vi "ap2 (hw4).vi"() -> ()   [LabVIEW 2017]
panel:
  in  "Stop":bool
  out "Equation used":string
  out "Result":dbl
  in  "Operation":T1(ring)
  in  "Y":dbl
  in  "X":dbl
  # "AP2"
  # "Patrik Sokolowski"
  # "In order to update the result after changing the Operation,   change the X or Y."
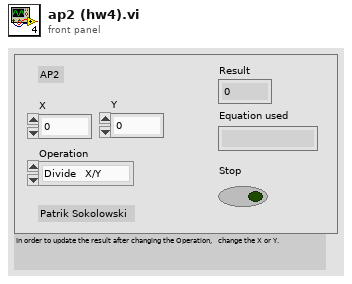
[diagram p1: front panel]
types:
  T1 = enum16{"Divide   X/Y", "Multiply   X*Y", "Subtract   X-Y", "Add   X+Y"}
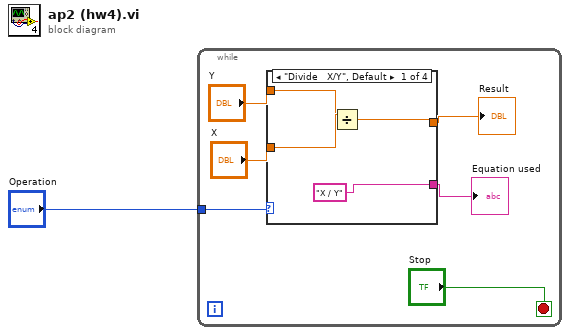
[diagram p0: block diagram]
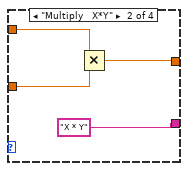
[diagram p2: hidden frame]
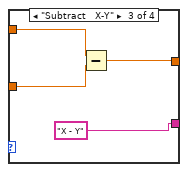
[diagram p3: hidden frame]
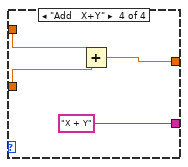
[diagram p4: hidden frame]
diagram:
  n1 = while {
    tunnel: "Operation" -> [w7]
    stop <- "Stop" stop-if-true
    n2 = case shown="\"Divide   X/Y\", Default" w7 {
      tunnel: [w9 w13 w17 w23] -> w4
      tunnel: "X" -> [w11 w15 w19 w22]
      tunnel: "Y" -> [w10 w14 w18 w21]
      tunnel: ["X / Y" "X * Y" "X - Y" "X + Y"] -> w3
      frame "Divide   X/Y", Default {
        n3 = Divide(x=w11, y=w10) -> (x/y=w9:dbl)
      }
      frame "Multiply   X*Y" {
        n4 = Multiply(x=w14, y=w15) -> (x*y=w13:dbl)
      }
      frame "Subtract   X-Y" {
        n5 = Subtract(x=w18, y=w19) -> (x-y=w17:dbl)
      }
      frame "Add   X+Y" {
        n6 = Add(x=w22, y=w21) -> (x+y=w23:dbl)
      }
    }
    "Result" <- w4
    "Equation used" <- w3
  }
